vi "auto phase nanonis.vi"(0 "Num averages":u32) -> ()   [LabVIEW 2021]
uses:
  <userlib>/Nanonis Prog Interface V5/Nanonis Prog Interface.lvlib
panel:
  out "arctan(x)":sgl
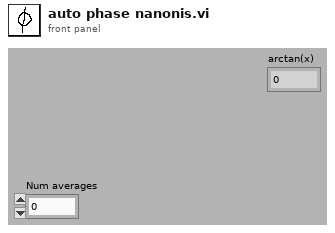
[diagram p1: front panel]
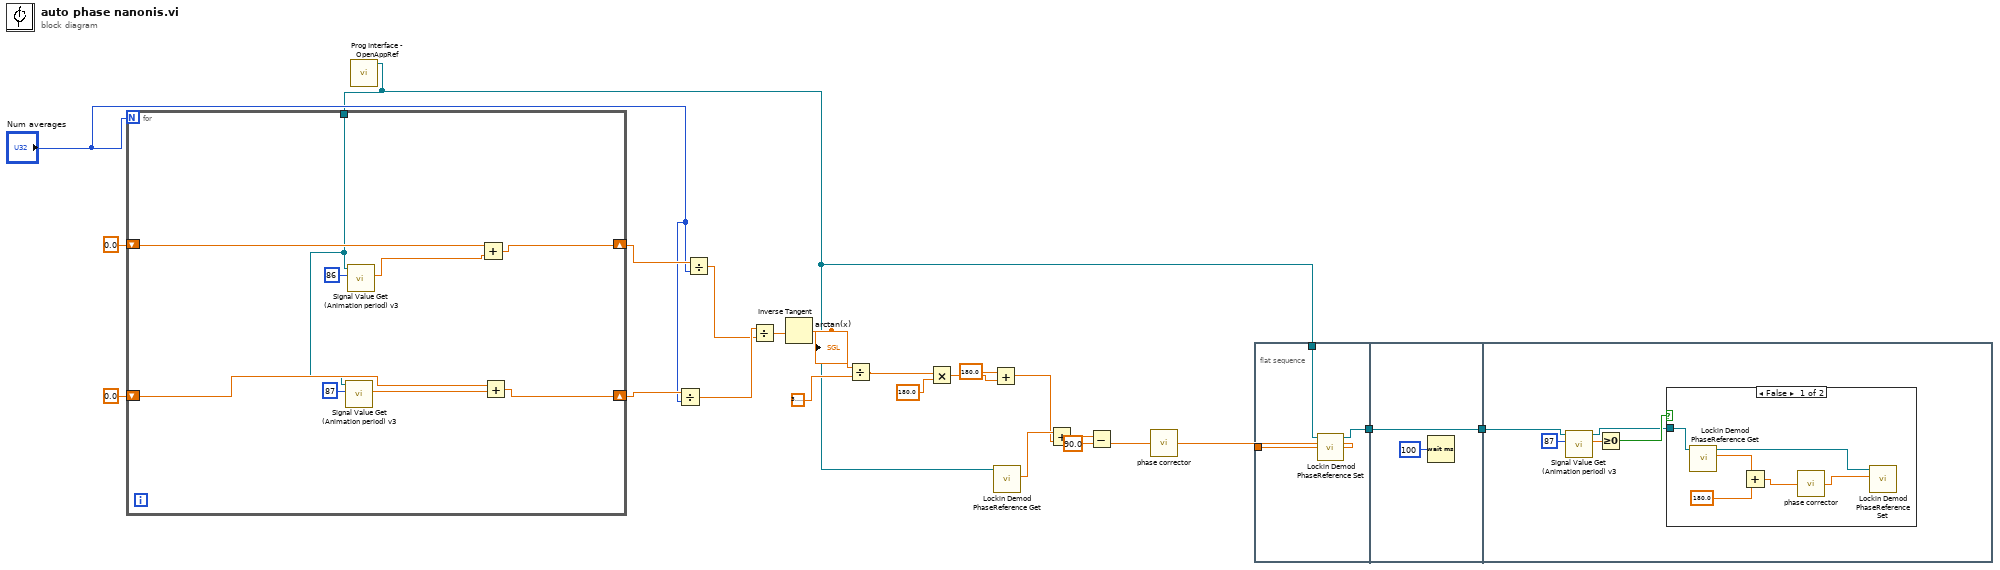
[diagram p0: block diagram]
diagram:
  n1 = call <userlib>:"Prog Interface - OpenAppRef.vi"() -> ("Application reference"=w3:refnum<vi>)  [unwired: 6 in, 1 out]
  n2 = for {
    N: "Num averages" -> [_]
    shift-right: [w29] -> w23
    shift-left: sgl 0.0 -> [w30]
    shift-right: [w26] -> w22
    shift-left: sgl 0.0 -> [w25]
    tunnel: w3 -> [w24]
    n3 = call <userlib>:"Signal Value Get (Animation period) v3.vi"("Signal index (0-127)"=i8 87, "Application ref in"=w24) -> ("Signal value"=w27:sgl)  [unwired: 6 in, 2 out]
    n4 = call <userlib>:"Signal Value Get (Animation period) v3.vi"("Signal index (0-127)"=i8 86, "Application ref in"=w24) -> ("Signal value"=w31:sgl)  [unwired: 6 in, 2 out]
    n5 = Add(x=w30, y=w31) -> (x+y=w29:sgl)
    n6 = Add(x=w25, y=w27) -> (x+y=w26:sgl)
  }
  n7 = Divide(x=w22, y="Num averages") -> (x/y=w19:sgl)
  n8 = Divide(x=w23, y="Num averages") -> (x/y=w18:sgl)
  n9 = Divide(x=w19, y=w18) -> (x/y=w20:sgl)
  n10 = Inverse Tangent(1:w20) -> (0:w17:sgl)
  "arctan(x)" <- w17
  n11 = Divide(x=w17, y=3.141592653589793) -> (x/y=w8:dbl)
  n12 = Multiply(x=w8, y=180.0) -> (x*y=w13:dbl)
  n13 = Add(x=180.0, y=w13) -> (x+y=w10:dbl)
  n14 = call <userlib>:"Lockin Demod PhaseReference Get.vi"("Application ref in"=w3) -> ("Phase Reference"=w14:sgl)  [unwired: 8 in, 2 out]
  n15 = Add(x=w14, y=w10) -> (x+y=w7:dbl)
  n16 = Subtract(x=w7, y=90.0) -> (x-y=w5:dbl)
  n17 = call "phase corrector.vi"("Phase"=w5) -> ("Corrected phase"=w4:dbl)
  n18 = flat-sequence {
    tunnel: w4 -> [w35]
    tunnel: w3 -> [w34]
    tunnel: [w33] -> w2
    tunnel: w2 -> [w37]
    tunnel: [w37] -> w1
    tunnel: w1 -> [w39]
    frame #0 {
      n19 = call <userlib>:"Lockin Demod PhaseReference Set.vi"("Phase Reference"=w35, "Application ref in"=w34) -> ("Application ref out"=w33:refnum<vi>)  [unwired: 8 in, 1 out]
    }
    frame #1 {
      n20 = Wait (ms)(milliseconds to wait=u32 100) -> ()  [unwired: 1 out]
    }
    frame #2 {
      n21 = call <userlib>:"Signal Value Get (Animation period) v3.vi"("Signal index (0-127)"=i8 87, "Application ref in"=w39) -> ("Signal value"=w41:sgl, "Application ref out"=w38:refnum<vi>)  [unwired: 6 in, 1 out]
      n22 = Greater Or Equal To 0?(x=w41) -> (x >= 0?=w40:bool)
      n23 = case shown="False" w40 {
        tunnel: w38 -> [w44 _]
        frame False {
          n24 = call <userlib>:"Lockin Demod PhaseReference Get.vi"("Application ref in"=w44) -> ("Phase Reference"=w48:sgl, "Application ref out"=w43:refnum<vi>)  [unwired: 8 in, 1 out]
          n25 = Add(x=w48, y=sgl 180.0) -> (x+y=w46:sgl)
          n26 = call "phase corrector.vi"("Phase"=w46) -> ("Corrected phase"=w45:dbl)
          n27 = call <userlib>:"Lockin Demod PhaseReference Set.vi"("Phase Reference"=w45, "Application ref in"=w43) -> ()  [unwired: 8 in, 2 out]
        }
        frame True {
        }
      }
    }
  }
